vi "hyst_sat_drift_cascade_parallel.vi"(4 "N_hyst":i32, 6 "N_sat":i32, 7 "parallel_inv":bool=TRUE, 8 "Den":sgl[](array[numeric])=[0.982758, -1.98194, 1.0, 0.0, 0.0, 0.0, 0.0, 0.0, 0.0], 9 "Num":sgl[](array[numeric])=[-0.00254, 0.000408, 0.00295, 0.0, 0.0, 0.0, 0.0, 0.0, 0.0], 10 "TF Order":i32=2, 11 "u_k (un saturated)":fxp<+/-,32,5>) -> (2 "Hinv(uk)":fxp<+/-,32,10>)   [LabVIEW 2017]
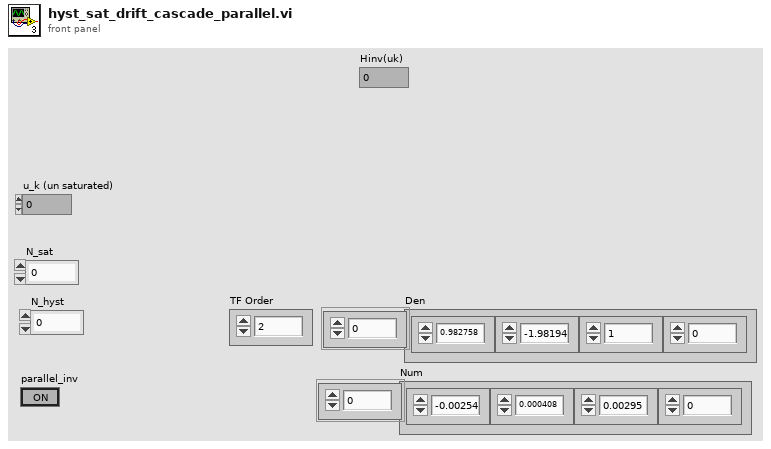
[diagram p1: front panel]
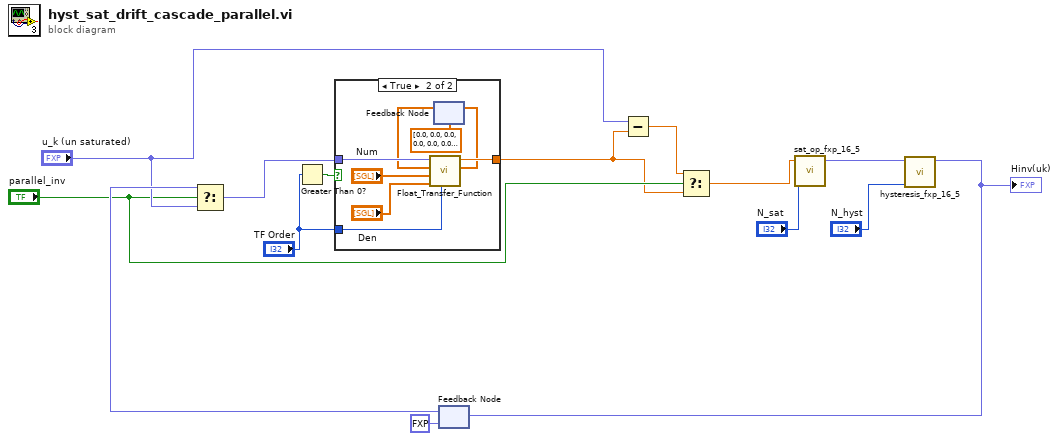
[diagram p0: block diagram]
diagram:
  n1 = Greater Than 0?(x="TF Order") -> (x > 0?=w10:bool)
  n2 = feedback #1(fxp<+/-,32,10> 0.0 ("Hinv(uk)")) -> (w7:fxp<+/-,32,10>)
  n3 = Select(t=w7, s="parallel_inv", f="u_k (un saturated)") -> (s? t:f=w8:fxp<+/-,37,10>)
  n4 = case shown="True" w10 {
    tunnel: w8 -> [w15 w23]
    tunnel: "TF Order" -> [_ w22]
    tunnel: [w15 w21] -> w2
    frame False {
    }
    frame True {
      n5 = feedback #2(sgl[] [0.0, 0.0, 0.0, 0.0, 0.0, 0.0, 0.0, 0.0, 0.0] ("State Out")) -> (w19:sgl[])
      n6 = call "Float_Transfer_Function.vi"("TF Order"=w22, "Den"="Den", "Num"="Num", "State In"=w19, "Input"=w23) -> ("State Out"=w20:sgl[], "Output"=w21:sgl)  [unwired: 4 in]
      n7 = feedback-in #2(w20) -> ()
    }
  }
  n8 = Subtract(x="u_k (un saturated)", y=w2) -> (x-y=w3:sgl)
  n9 = Select(t=w3, s="parallel_inv", f=w2) -> (s? t:f=w4:sgl)
  n10 = call "sat_op_fxp_16_5.vi"("N_sat"="N_sat", "uk_in"=w4) -> ("Hinv(uk)"=w14:fxp<+/-,32,10>)  [unwired: 9 in]
  n11 = call "hysteresis_fxp_16_5.vi"("N_hyst"="N_hyst", "uk_in"=w14) -> ("Hinv(uk)"=w11:fxp<+/-,32,10>)  [unwired: 9 in]
  "Hinv(uk)" <- w11
  n12 = feedback-in #1(w11) -> ()
